vi "Send move to stage.vi"(8 "error in (no error)":errorcluster, 10 "move to send":dbl[unit], 11 "Retiga in":refnum<class "Retiga.lvclass">) -> (0 "error out":errorcluster, 3 "Retiga out":refnum<class "Retiga.lvclass">)   [LabVIEW 2012, in "Retiga.lvclass"]
uses:
  Retiga.lvclass
  <vilib>/Distrio/Murmex/GenericMessage/GenericMessage.lvclass
  Retiga.lvclass/Retiga.ctl
  <vilib>/Distrio/Murmex/Message/Message.lvclass
  <vilib>/Distrio/Murmex/Murmex/Murmex.lvclass
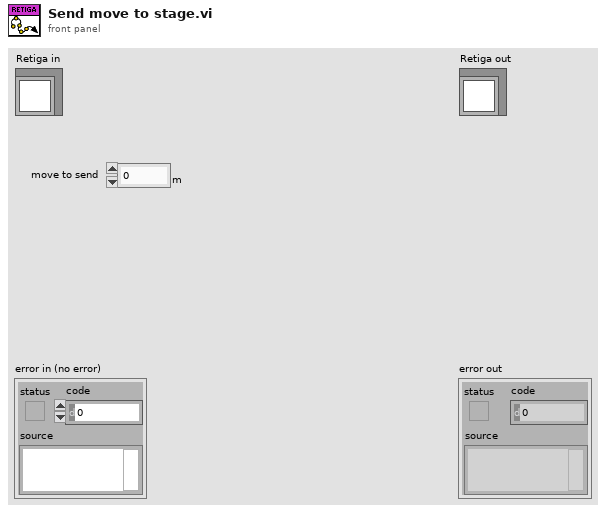
[diagram p1: front panel]
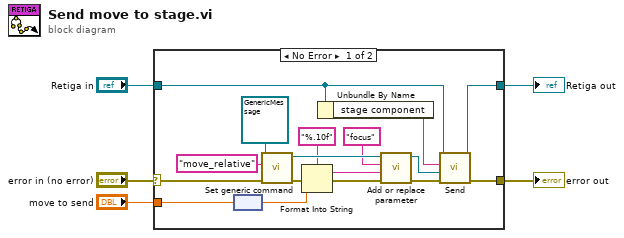
[diagram p0: block diagram]
diagram:
  n1 = case shown="No Error" "error in (no error)" {
    selector: "error in (no error)" -> [w10 w24]
    tunnel: [w9 w24] -> w4
    tunnel: [w11 w23] -> w2
    tunnel: "Retiga in" -> [w12 w23]
    tunnel: "move to send" -> [w7 _]
    frame No Error {
      n2 = node(w7) -> (w8:dbl)
      n3 = call <vilib>:"Set generic command.vi"("error in (no error)"=w10, "generic command"="move_relative" ("command string"), "GenericMessage in"=refnum<class "GenericMessage.lvclass"> refnum ("Murmex.lvlib:GenericMessage")) -> ("error out"=w19:errorcluster, "GenericMessage out"=w22:refnum<class "GenericMessage.lvclass">)  [unwired: 7 in]
      n4 = Format Into String(format string="%.10f", error in=w19, w8) -> (resulting string=w17:string, error out=w18:errorcluster)  [unwired: 1 in]
      n5 = Unbundle By Name(w12) -> ("stage component"=w13:string)
      n6 = call <vilib>:"Add or replace parameter.vi"("error in (no error)"=w18, "value"=w17, "name"="focus", "Message in"=w22) -> ("error out"=w20:errorcluster, "Message out"=w21:refnum<class "GenericMessage.lvclass">)  [unwired: 6 in]
      n7 = call <vilib>:"Send.vi"("error in (no error)"=w20, "Message"=w21, "recipient"=w13, "Murmex in"=w12) -> ("error out"=w9:errorcluster, "Murmex out"=w11:refnum<class "Retiga.lvclass">)  [unwired: 6 in]
    }
    frame Error {
    }
  }
  "error out" <- w4
  "Retiga out" <- w2
